vi "Vision Server.vi"(8 "error in":errorcluster, 11 "port":u16=8254) -> (0 "error out":errorcluster)   [LabVIEW 2016, in "Vision Server.lvclass"]
uses:
  Vision Server.lvclass
  typedef/Message Type.ctl
  Vision Server.lvclass/Vision Server.ctl
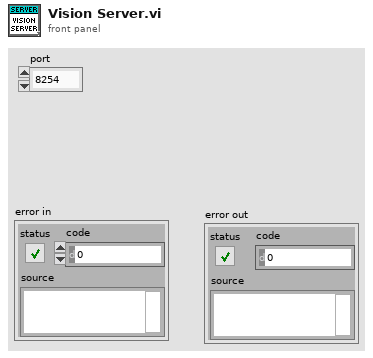
[diagram p1: front panel]
types:
  T1 = typedef "Vision Server.lvclass/Message Type.ctl" = cluster{"type":string, "message":string}
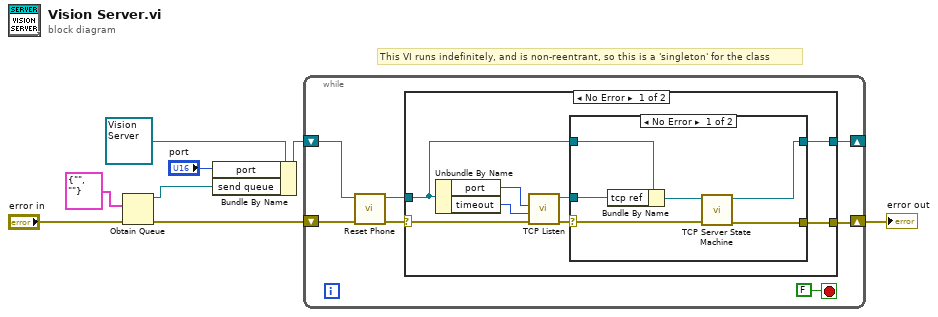
[diagram p0: block diagram]
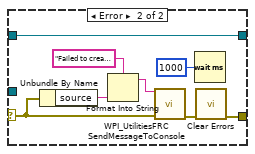
[diagram p2: hidden frame]
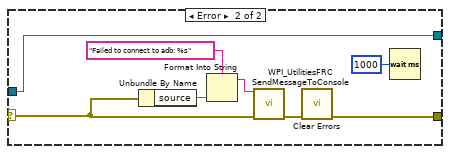
[diagram p3: hidden frame]
diagram:
  # "This VI runs indefinitely, and is non-reentrant, so this is a 'singleton' for the class"
  n1 = Obtain Queue(element data type=T1 {"type"="", "message"=""} ("Cluster"), error in (no error)="error in") -> (queue out=w4:refnum<queue>, error out=w2:errorcluster)  [unwired: 3 in, 1 out]
  n2 = Bundle By Name(cluster=refnum<class "Vision Server.lvclass"> refnum ("Vision Server.lvclass"), "port"="port", "send queue"=w4) -> (w1:refnum<class "Vision Server.lvclass">)
  n3 = while {
    shift-right: [w13] -> w8
    shift-left: w2 -> [w12]
    shift-right: [w14] -> _
    shift-left: w1 -> [w10]
    stop <- FALSE stop-if-true
    n4 = call "Reset Phone.vi"("error in (no error)"=w12, "Vision Server in"=w10) -> ("error out"=w11:errorcluster, "Vision Server out"=w9:refnum<class "Vision Server.lvclass">)  [unwired: 8 in]
    n5 = case shown="No Error" w11 {
      selector: w11 -> [w18 w39]
      tunnel: [w20 w45] -> w14
      tunnel: [w19 w38] -> w13
      tunnel: w9 -> [w17 w45]
      frame No Error {
        n6 = Unbundle By Name(w17) -> ("port"=w22:u16, "timeout"=w16:i32)
        n7 = call <vilib>:"TCP Listen.vi"("error in (no error)"=w18, "timeout ms (wait forever: -1)"=w16, "port"=w22) -> ("error out"=w23:errorcluster, "connection ID"=w21:refnum<k5>)  [unwired: 4 in, 3 out]
        n8 = case shown="No Error" w23 {
          selector: w23 -> [w29 w30]
          tunnel: [w28 w31] -> w19
          tunnel: [w27 w37] -> w20
          tunnel: w17 -> [w26 w37]
          tunnel: w21 -> [w24 _]
          frame No Error {
            n9 = Bundle By Name(cluster=w26, "tcp ref"=w24) -> (w25:refnum<class "Vision Server.lvclass">)
            n10 = call "TCP Server State Machine.vi"("error in"=w29, "Vision Server in"=w25) -> ("error out"=w28:errorcluster, "Vision Server out"=w27:refnum<class "Vision Server.lvclass">)  [unwired: 8 in]
          }
          frame Error {
            n11 = Unbundle By Name(w30) -> ("source"=w34:string)
            n12 = Format Into String(format string="Failed to create server: %s", w34) -> (resulting string=w32:string)  [unwired: 2 in, 1 out]
            n13 = call <vilib>:"WPI_UtilitiesFRC SendMessageToConsole.vi"("Message"=w32, "error in (no error)"=w30) -> ("error out"=w35:errorcluster)  [unwired: 13 in]
            n14 = Wait (ms)(milliseconds to wait=u32 1000) -> ()  [unwired: 1 out]
            n15 = call <vilib>:"Clear Errors.vi"("error in (no error)"=w35) -> ("error out"=w31:errorcluster)  [unwired: 5 in, 1 out]
          }
        }
      }
      frame Error {
        n16 = Unbundle By Name(w39) -> ("source"=w43:string)
        n17 = Format Into String(format string="Failed to connect to adb: %s", w43) -> (resulting string=w41:string)  [unwired: 2 in, 1 out]
        n18 = call <vilib>:"WPI_UtilitiesFRC SendMessageToConsole.vi"("Message"=w41, "error in (no error)"=w39) -> ("error out"=w40:errorcluster)  [unwired: 13 in]
        n19 = call <vilib>:"Clear Errors.vi"("error in (no error)"=w40) -> ("error out"=w38:errorcluster)  [unwired: 5 in, 1 out]
        n20 = Wait (ms)(milliseconds to wait=u32 1000) -> ()  [unwired: 1 out]
      }
    }
  }
  "error out" <- w8
